vi "Keithley 2400 Average Measure.vi"(7 "Measurement":enum16{"Voltage", "Current"}(ring), 8 "error in (no error)":errorcluster, 9 "Time per Point (ms)":u32, 10 "Points to Average":i32, 11 "VISA SR 7265":refnum<visa-resource-name>) -> (0 "error out":errorcluster, 3 "Measurement Array Out":dbl[](array[numeric]))   [LabVIEW 2019]
uses:
  <vilib>/Analysis/NI_AALBase.lvlib
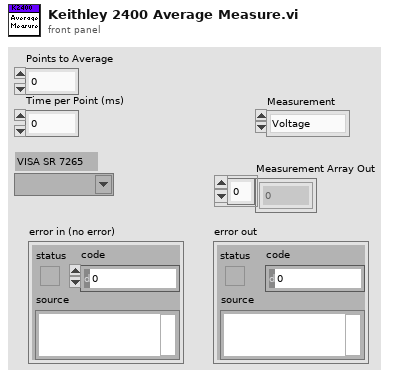
[diagram p1: front panel]
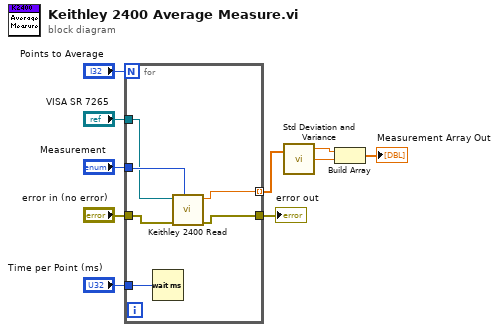
[diagram p0: block diagram]
diagram:
  n1 = for {
    N: "Points to Average" -> [_]
    tunnel: "error in (no error)" -> [w15]
    tunnel: "Time per Point (ms)" -> [w16]
    tunnel: "VISA SR 7265" -> [w12]
    tunnel: "Measurement" -> [w13]
    tunnel: [w11] -> w2 mode=indexing
    tunnel: [w14] -> w1
    n2 = Wait (ms)(milliseconds to wait=w16) -> ()  [unwired: 1 out]
    n3 = call "Keithley 2400 Read.vi"("Read Type"=w13, "error in (no error)"=w15, "VISA Refnum in"=w12) -> ("error out"=w14:errorcluster, "Voltage Reading"=w11:dbl)  [unwired: 7 in]
  }
  "error out" <- w1
  n4 = call <vilib>:"Std Deviation and Variance.vi"("X"=w2) -> ("mean"=w7:dbl, "standard deviation"=w8:dbl)  [unwired: 1 in, 1 out]
  n5 = Build Array(w7, w8) -> (→"Measurement Array Out":dbl[])
